vi "REPORT.BIN TO STRING.vi"(7 "Resultado test":bool) -> (8 "OK, Fault":string)   [LabVIEW 2019]
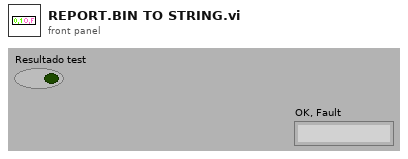
[diagram p1: front panel]
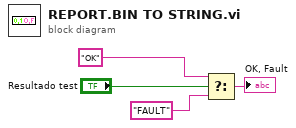
[diagram p0: block diagram]
diagram:
  n1 = Select(t="OK" ("OK o Fault"), s="Resultado test", f="FAULT") -> (s? t:f=→"OK, Fault":string)
